vi "LabJackToTemp.vi"(10 "LJ Data":dbl[](array[numeric]), 11 "File Path":path=path "C:/Xe") -> (3 "Temperatures":dbl[](array[numeric]))   [LabVIEW 2012]
uses:
  <vilib>/addons/h5labview2/file/H5Fmode.ctl
  <vilib>/addons/h5labview2/file/H5F.lvlib
  <vilib>/addons/h5labview2/dataset/H5D.lvlib
panel:
  # "This function converts the values read from addS-go-get\ninto an array of temperatures. They are indexed in order:\n0 - Time, 1 - RTD0, 2 - RTD1, 3 - RTD2, 4 - RTD3, 5 - RTD4\nIt also saves these values to the specified file."
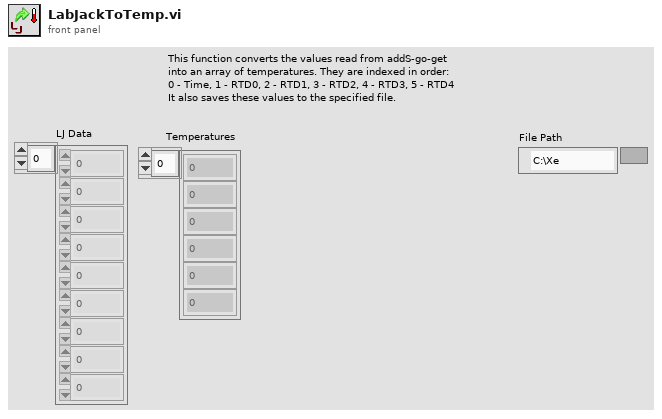
[diagram p1: front panel]
types:
  T1 = typedef "H5F.lvlib/H5Fmode.ctl" = enum16{"read-only", "read-write", "overwrite", "create new", "open or create"}
  T2 = typedef "hid_t.ctl" = i64
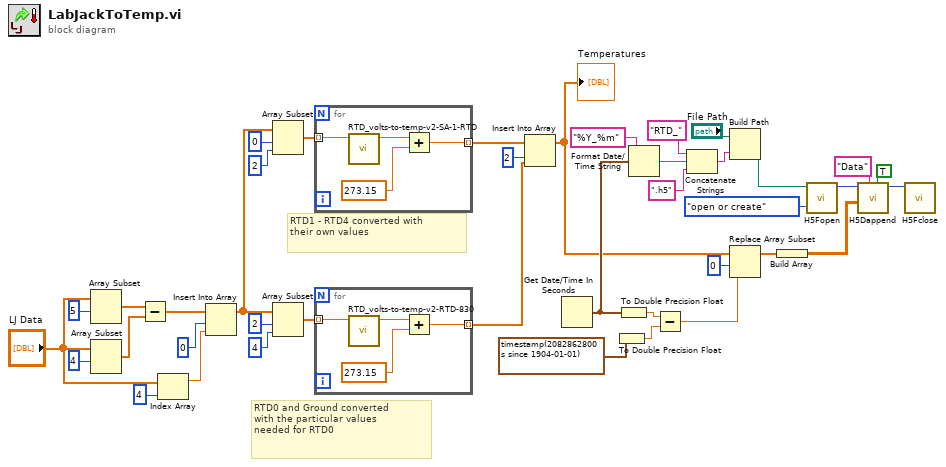
[diagram p0: block diagram]
diagram:
  # "RTD1 - RTD4 converted with\ntheir own values"
  # "RTD0 and Ground converted\nwith the particular values \nneeded for RTD0"
  n1 = Array Subset(array="LJ Data", index=5 ("Index")) -> (w35:dbl[])  [unwired: 1 in]
  n2 = Array Subset(array="LJ Data", index=4 ("Index")) -> (w37:dbl[])  [unwired: 1 in]
  n3 = Subtract(x=w35, y=w37) -> (x-y=w34:dbl[])
  n4 = Index Array(array="LJ Data", index=4) -> (element=w31:dbl)
  n5 = Insert Into Array(array=w34, index=0 ("Index"), new element=w31) -> (w23:dbl[])
  n6 = Array Subset(array=w23, index=0, length=2) -> (w27:dbl[])
  n7 = Array Subset(array=w23, index=2, length=4) -> (w24:dbl[])
  n8 = for {
    tunnel: [w43] -> w30 mode=indexing
    tunnel: w27 -> [w41] mode=indexing
    n9 = call "RTD_volts-to-temp-v2-SA-1-RTD.vi"("RTD Volts"=w41) -> ("Temp"=w42:dbl)  [unwired: 10 in]
    n10 = Add(x=w42, y=273.15) -> (x+y=w43:dbl)
  }
  n11 = for {
    tunnel: [w47] -> w39 mode=indexing
    tunnel: w24 -> [w45] mode=indexing
    n12 = call "RTD_volts-to-temp-v2-RTD-830.vi"("RTD Volts"=w45) -> ("Temp"=w46:dbl)  [unwired: 10 in]
    n13 = Add(x=w46, y=273.15) -> (x+y=w47:dbl)
  }
  n14 = Insert Into Array(array=w30, index=2 ("Index"), new element=w39) -> (w1:dbl[])
  "Temperatures" <- w1
  n15 = Get Date/Time In Seconds() -> (seconds since 1Jan1904=w7:timestamp)
  n16 = To Double Precision Float(number=timestamp(2082862800 s since 1904-01-01)) -> (double precision float=w11:dbl)
  n17 = To Double Precision Float(number=w7) -> (double precision float=w12:dbl)
  n18 = Format Date/Time String(time format string (%c)="%Y_%m", seconds (now)=w7) -> (date/time string=w6:string)  [unwired: 1 in]
  n19 = Subtract(x=w12, y=w11) -> (x-y=w10:dbl)
  n20 = Concatenate Strings("RTD_" ("string"), w6, ".h5" ("string")) -> (w4:string)
  n21 = Build Path(base path="File Path", name or relative path=w4) -> (appended path=w3:path)
  n22 = Replace Array Subset(array=w1, new element=w10, index=0) -> (w20:dbl[])
  n23 = Build Array(w20) -> (w19:dbl[][])
  n24 = call <vilib>:"H5Fopen.vi"("mode (read-only)"=H5Fmode."open or create", "path"=w3) -> ("ref out"=w16:T2)  [unwired: 8 in, 1 out]
  n25 = call <vilib>:"H5Dappend.vi"("create? (T)"=TRUE, "dataset name"="Data", "data"=w19, "ref in"=w16) -> ("ref out"=w15:T2)  [unwired: 4 in, 3 out]
  n26 = call <vilib>:"H5Fclose.vi"("ref"=w15) -> ()  [unwired: 10 in, 1 out]
